vi "Test_Exe_Build VI.vi"() -> ()   [LabVIEW 2020]
uses:
  <vilib>/AppBuilder/AB_API_Simple/Build Specification Version.ctl
  <vilib>/AppBuilder/AB_API_Simple/Get Build Specification Version (path).vi
  <vilib>/AppBuilder/AB_API_Simple/Set Build Specification Version (path).vi
  <vilib>/AppBuilder/AB_API_Simple/NI_App_Builder_API.lvlib
panel:
  in  "Build Specification Version to set":T1
  out "error out":errorcluster
  out "Build Specification Version":T1
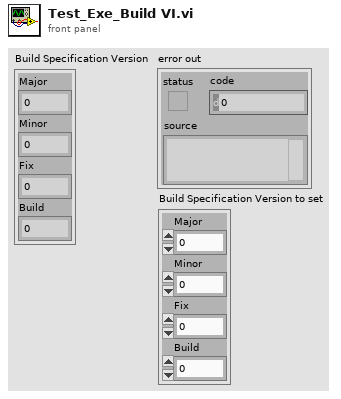
[diagram p1: front panel]
types:
  T1 = typedef "NI_App_Builder_API.lvlib/Build Specification Version.ctl" = cluster{"Major":u16, "Minor":u16, "Fix":u16, "Build":u16}
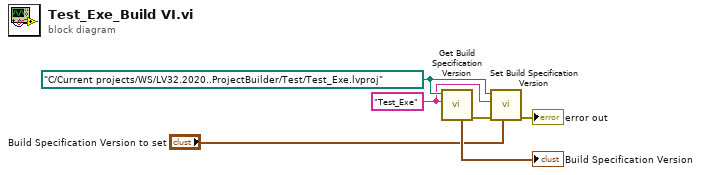
[diagram p0: block diagram]
diagram:
  w2 = "Test_Exe" ("Name of build specification")
  w3 = path "C:/Current projects/WS/LV32.2020..ProjectBuilder/Test/Test_Exe.lvproj" ("Path to project")
  n1 = call-poly <vilib>:"Get Build Specification Version.vi"("Name of build specification"=w2, "Path to project"=w3) -> ("error out"=w5:errorcluster, "Build Specification Version"=→"Build Specification Version":T1)  [unwired: 8 in]
  n2 = call-poly <vilib>:"Set Build Specification Version.vi"("Build Specification Version"="Build Specification Version to set", "error in (no error)"=w5, "Name of build specification"=w2, "Path to project"=w3) -> ("error out"=→"error out":errorcluster)  [unwired: 7 in]
